vi "ZMQ GEECS subscriber.vi"() -> ()   [LabVIEW 2020]
uses:
  <vilib>/addons/zeromq/socket_type.ctl
  <vilib>/addons/zeromq/socket_options.ctl
  <vilib>/addons/zeromq/zmq_context.lvclass
  <vilib>/addons/zeromq/zeromq.lvlib
  <vilib>/addons/zeromq/zmq_socket.lvclass
panel:
  out "Waveform Chart":i32(graph)
  out "timeout?":bool
  in  "endpoint":string="tcp://192.168.14.2:" caption="endpoint (publisher IP)"
  out "error out":errorcluster
  in  "Stop":bool
  in  "ports":i32[](array[numeric])=[5555, 5556, 5557]
  out "messages":string[](array[string])
  # "ZeroMQ subscriber VI"
  # "Subscribe to all messages published to specified ports"
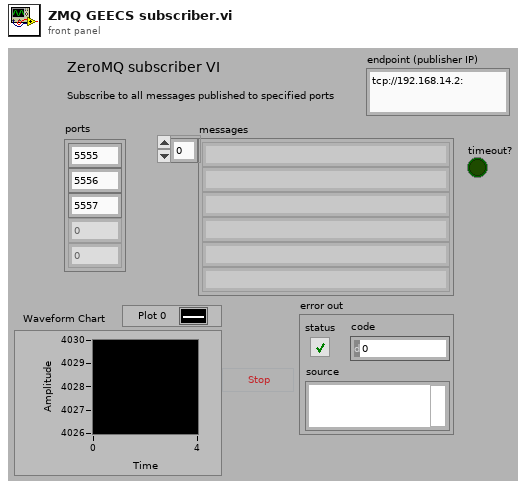
[diagram p1: front panel]
types:
  T1 = typedef "zeromq.lvlib/socket_options.ctl" = enum8{"NONE", "ZMQ_HWM", "<2>", "ZMQ_SWAP", "ZMQ_AFFINITY", "ZMQ_ROUTING_ID", "ZMQ_SUBSCRIBE", "ZMQ_UNSUBSCRIBE", "ZMQ_RATE", "ZMQ_RECOVERY_IVL", "ZMQ_MCAST_LOOP", "ZMQ_SNDBUF", "ZMQ_RCVBUF", "ZMQ_RCVMORE", "ZMQ_FD", "ZMQ_EVENTS", "ZMQ_TYPE", "ZMQ_LINGER", "ZMQ_RECONNECT_IVL", "ZMQ_BACKLOG", "ZMQ_RECOVERY_IVL_MSEC", "ZMQ_RECONNECT_IVL_MAX", "ZMQ_MAXMSGSIZE", "ZMQ_SNDHWM", "ZMQ_RCVHWM", "ZMQ_MULTICAST_HOPS", "<26>", "ZMQ_RCVTIMEO", "ZMQ_SNDTIMEO", "<29>", "<30>", "ZMQ_IPV4ONLY", "ZMQ_LAST_ENDPOINT", "ZMQ_ROUTER_MANDATORY", "ZMQ_TCP_KEEPALIVE", "ZMQ_TCP_KEEPALIVE_CNT", "ZMQ_TCP_KEEPALIVE_IDLE", "ZMQ_TCP_KEEPALIVE_INTVL", "ZMQ_TCP_ACCEPT_FILTER", "ZMQ_IMMEDIATE", "ZMQ_XPUB_VERBOSE", "ZMQ_ROUTER_RAW", "ZMQ_IPV6", "ZMQ_MECHANISM", "ZMQ_PLAIN_SERVER", "ZMQ_PLAIN_USERNAME", "ZMQ_PLAIN_PASSWORD", "ZMQ_CURVE_SERVER", "ZMQ_CURVE_PUBLICKEY", "ZMQ_CURVE_SECRETKEY", "ZMQ_CURVE_SERVERKEY", "ZMQ_PROBE_ROUTER", "ZMQ_REQ_CORRELATE", "ZMQ_REQ_RELAXED", "ZMQ_CONFLATE", "ZMQ_ZAP_DOMAIN", "ZMQ_ROUTER_HANDOVER", "ZMQ_TOS", "ZMQ_IPC_FILTER_PID", "ZMQ_IPC_FILTER_UID", "ZMQ_IPC_FILTER_GID", "ZMQ_CONNECT_ROUTING_ID", "ZMQ_GSSAPI_SERVER", "ZMQ_GSSAPI_PRINCIPAL", "ZMQ_GSSAPI_SERVICE_PRINCIPAL", "ZMQ_GSSAPI_PLAINTEXT", "ZMQ_HANDSHAKE_IVL", "<67>", "ZMQ_SOCKS_PROXY", "ZMQ_XPUB_NODROP", "ZMQ_BLOCKY", "ZMQ_XPUB_MANUAL", "ZMQ_XPUB_WELCOME_MSG", "ZMQ_STREAM_NOTIFY", "ZMQ_INVERT_MATCHING", "ZMQ_HEARTBEAT_IVL", "ZMQ_HEARTBEAT_TTL", "ZMQ_HEARTBEAT_TIMEOUT", "ZMQ_XPUB_VERBOSER", "ZMQ_CONNECT_TIMEOUT", "ZMQ_TCP_MAXRT", "ZMQ_THREAD_SAFE", "<82>", "<83>", "ZMQ_MULTICAST_MAXTPDU", "ZMQ_VMCI_BUFFER_SIZE", "ZMQ_VMCI_BUFFER_MIN_SIZE", "ZMQ_VMCI_BUFFER_MAX_SIZE", "ZMQ_VMCI_CONNECT_TIMEOUT", "ZMQ_USE_FD", "ZMQ_GSSAPI_PRINCIPAL_NAMETYPE", "ZMQ_GSSAPI_SERVICE_PRINCIPAL_NAMETYPE", "ZMQ_BINDTODEVICE", "ZMQ_ZAP_ENFORCE_DOMAIN", "ZMQ_LOOPBACK_FASTPATH", "ZMQ_METADATA", "ZMQ_MULTICAST_LOOP", "ZMQ_ROUTER_NOTIFY"}
  T2 = typedef "zeromq.lvlib/socket_type.ctl" = enum8{"ZMQ_PAIR", "ZMQ_PUB", "ZMQ_SUB", "ZMQ_REQ", "ZMQ_REP", "ZMQ_DEALER", "ZMQ_ROUTER", "ZMQ_PULL", "ZMQ_PUSH", "ZMQ_XPUB", "ZMQ_XSUB", "ZMQ_STREAM", "ZMQ_SERVER", "ZMQ_CLIENT", "ZMQ_RADIO", "ZMQ_DISH", "ZMQ_GATHER", "ZMQ_SCATTER", "ZMQ_DGRAM"}
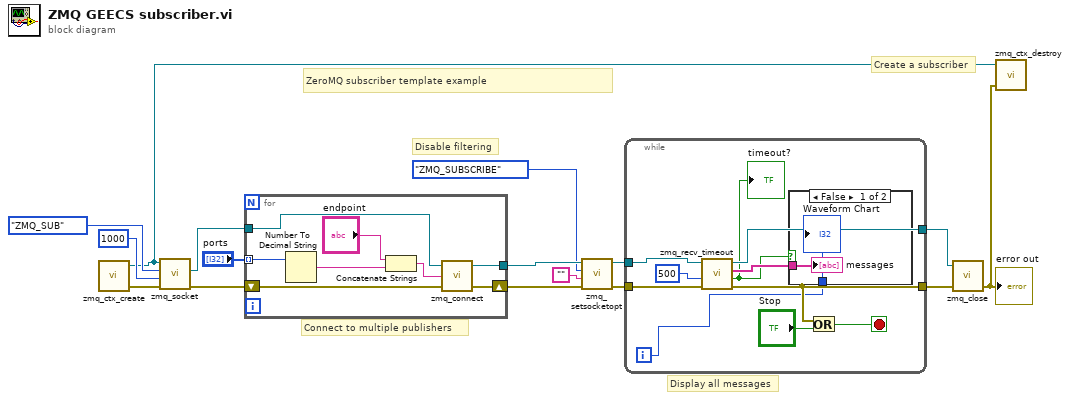
[diagram p0: block diagram]
diagram:
  # "ZeroMQ subscriber template example"
  # "Display all messages"
  # "Create a subscriber"
  # "Disable filtering"
  # "Connect to multiple publishers"
  n1 = call <vilib>:"zmq_ctx_create.vi"() -> ("error out"=w15:errorcluster, "context out"=w5:refnum<class "zmq_context.lvclass">)  [unwired: 4 in]
  n2 = call <vilib>:"zmq_socket.vi"("error in"=w15, "linger (ms)"=1000, "socket type"=socket_type."ZMQ_SUB", "context in"=w5) -> ("error out"=w14:errorcluster, "socket out"=w7:refnum<class "zmq_socket.lvclass">)  [unwired: 1 in, 1 out]
  n3 = for {
    tunnel: w7 -> [w24]
    tunnel: [w21] -> w13
    tunnel: "ports" -> [w17] mode=indexing
    shift-right: [w20] -> w12
    shift-left: w14 -> [w23]
    n4 = Number To Decimal String(number=w17) -> (decimal integer string=w18:string)  [unwired: 1 in]
    n5 = Concatenate Strings("endpoint", w18) -> (w19:string)
    n6 = call <vilib>:"zmq_connect.vi"("error in"=w23, "endpoint"=w19, "socket in"=w24) -> ("error out"=w20:errorcluster, "socket out"=w21:refnum<class "zmq_socket.lvclass">)  [unwired: 1 in]
  }
  n7 = call <vilib>:"zmq_setsocketopt.vi"("error in"=w12, "value"="", "option"=socket_options."ZMQ_SUBSCRIBE", "socket in"=w13) -> ("error out"=w11:errorcluster, "socket out"=w4:refnum<class "zmq_socket.lvclass">)  [unwired: 2 in]
  n8 = while {
    tunnel: w4 -> [w34]
    tunnel: w11 -> [w33]
    tunnel: [w28] -> w2
    tunnel: [w29] -> w3
    i -> [w25]
    stop <- w30 stop-if-true
    n9 = call <vilib>:"zmq_recv_timeout.vi"("error in"=w33, "timeout (ms)"=u32 500, "socket in"=w34) -> ("error out"=w28:errorcluster, "timeout?"=w26:bool, "parts"=w27:string[], "socket out"=w29:refnum<class "zmq_socket.lvclass">)  [unwired: 1 in]
    "timeout?" <- w26
    n10 = case shown="False" w26 {
      tunnel: w27 -> [w36 _]
      tunnel: w25 -> [w35 _]
      frame False {
        "messages" <- w36
        "Waveform Chart" <- w35
      }
      frame True {
      }
    }
    n11 = Or(x=w28, y="Stop") -> (x .or. y?=w30:bool)
  }
  n12 = call <vilib>:"zmq_close.vi"("error in"=w2, "socket"=w3) -> ("error out"=w1:errorcluster)  [unwired: 3 in]
  "error out" <- w1
  n13 = call <vilib>:"zmq_ctx_destroy.vi"("error in"=w1, "context in"=w5) -> ()  [unwired: 3 in, 1 out]
